vi "re_LuaVIEW Pull (flat data).vi"(0 "default flat data":string, 2 "type descriptor":i16[](array[numeric]) format="%x", 5 "LuaVIEW reference in":T1, 11 "error in (no error)":errorcluster) -> (4 "flat data":string, 6 "LuaVIEW reference out":T1, 15 "error out":errorcluster)   [LabVIEW 2013]
doc: "Retrieves the item at the head/bottom of the Lua stack, translates it to a flat LabVIEW data string, and removes the item from the stack, thereby shifting any remaining data items down by one. Use this reentrant variant instead of the non-reentrant variant when pulling lots of flat data to prevent the non-reentrant VI from becoming contended. The most important use for this VI is to transfer compound data from Lua (a table) to LabVIEW (a cluster or array). To perform the translation, this function requires the type descriptor of the LabVIEW type/cluster/array that specifies how the translation is to take place. To use the flat data on the LabVIEW side, unflatten it.\n\nThe translation is recursive and thus handles nested clusters and arrays. If no translation is possible, e.g. because a LabVIEW array type is specified but no Lua table is provided, an error is returned. The LuaVIEW manual details which translations are supported.\n\nWhen the optional <B>default flat data</B> input is wired, its content will be used when either the Lua stack is empty or the Lua data item is nil. Note that allowing an empty stack is somewhat different from the other pull variants. It simplifies the implementation of an optional argument at the end of the argument list such that its omission causes the setting of default data.\n\nWhen default data is wired and the Lua data item has missing/nil table elements that map into a cluster element that is not inside an array, a partial substition of only these elements is performed so that the Lua-side data need not be fully specified. This is like a bundle by name where some cluster elements are not specified and the default data serves the role of the input cluster.\n\nThis VI is part of a polymorphic set that supports the pulling various data types. To change the type being pulled, pop up on this VI's diagram icon and use the \"Select Type\" sub menu."
uses:
  typedefs/t_LuaVIEW Reference.ctl
  typedefs/et_LuaVIEW CIN Actions.ctl
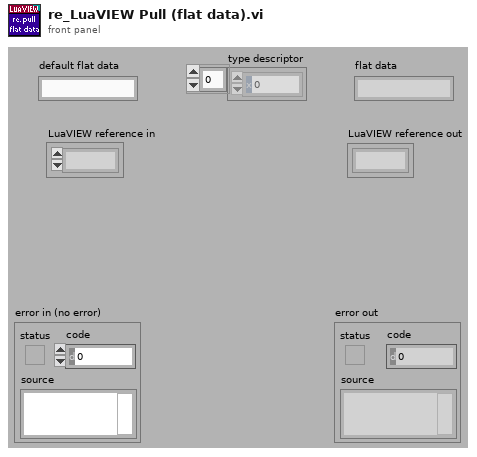
[diagram p1: front panel]
types:
  T1 = typedef "t_LuaVIEW Reference.ctl" = refnum<k1>
  T2 = typedef "et_LuaVIEW CIN Actions.ctl" = enum16{"checksynopsis", "_open", "_registerpublic", "_registerexport", "__never_an_error_result_ns", "luaversion", "cinversion", "_totals", "_taskcount", "pathological", "_unregnextpublic", "registryusecount", "__per_state_actions", "regsetprivate", "regsetindex", "regsetmodule", "_revokeexports", "_usepublic", "prepare", "compile", "execute", "call", "unregstaterefs", "_close", "pullboolean", "pullnumber", "pullI8", "pullU8", "pullI16", "pullU16", "pullI32", "pullU32", "pullobject", "pullrefnum", "pullstring", "pullflat", "pushflat", "pushobject", "getattribute", "setattribute", "stacktostring", "_startyieldtest", "_endyieldtest", "_pollprintbuffer", "__never_an_error_result_ps", "_pollexport", "setclone", "forcecleanup", "gettop", "clearstack", "insert", "pushboolean", "pushnumber", "pushrefnum", "pushstring", "pushnil", "pushvalue", "gettaskref", "settaskref"}
  T3 = typedef "et_LuaVIEW CIN Results.ctl" = enum16{"OK", "error", "main", "call", "clonecall", "modulecall", "exportcall", "index", "yield"}
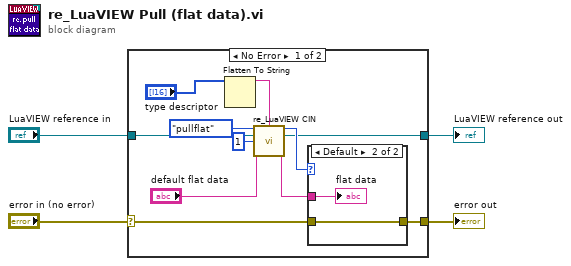
[diagram p0: block diagram]
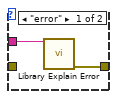
[diagram p2: hidden frame]
diagram:
  n1 = case shown="No Error" "error in (no error)" {
    selector: "error in (no error)" -> [w10 w21]
    tunnel: [w6 w20] -> w4
    tunnel: [w12 w21] -> w3
    tunnel: "LuaVIEW reference in" -> [w14 w20]
    frame No Error {
      n2 = Flatten To String(anything="type descriptor") -> (data string=w7:string)  [unwired: 3 in, 2 out]
      n3 = call "re_LuaVIEW CIN.vi"("action"=et_LuaVIEW_CIN_Actions."pullflat", "supplement"=w7, "LuaVIEW reference in"=w14, "index in"=1, "string in"="default flat data") -> ("result"=w13:T3, "LuaVIEW reference out"=w6:T1, "string out"=w11:string)  [unwired: 4 in, 4 out]
      n4 = case shown="Default" w13 {
        tunnel: [w17 w19] -> w12
        tunnel: w11 -> [w16 w18]
        tunnel: w10 -> [_ w19]
        frame "error" {
          n5 = call "Library Explain Error.vi"("explanation prefix (none)"=w16) -> ("explained error"=w17:errorcluster)  [unwired: 14 in]
        }
        frame Default {
          "flat data" <- w18
        }
      }
    }
    frame Error {
    }
  }
  "LuaVIEW reference out" <- w4
  "error out" <- w3
